vi "StateLED.vi"(0 "Master State":enum16{"Normal", "Climb"}(ring)) -> ()   [LabVIEW 2020]
doc: "This VI manages the apperance of the LEDs. The LED coloration and blink pattern report the robot mode and status. See project documentation for details."
uses:
  drivercommands.vi
  robotoutputs.vi
  driverdata.vi
  refnumbers.vi
  sensordata.vi
  autonomousinfo.vi
  <vilib>/vision/NI_Vision_Development_Module.lvlib
panel:
  in  "Color Sensor Raw Index":i32=44
  in  "Cowl Limit Reverse Index":i32=11
  in  "Turret Limit Forward Index":i32=9
  in  "Turret Limit Reverse Index":i32=8
  in  "Tower Sensor Index":i32=46
  in  "Boolean Sensor Off":u32(colorbox)=16750592
  in  "Boolean Sensor On":u32(colorbox)=6618880
  in  "Indexer Sensor Index":i32=45
  in  "Intaking":u32(colorbox)=16711692
  in  "Firing":u32(colorbox)=61212
  in  "Spinning":u32(colorbox)=16765440
  in  "User Value Choice":u8(slide)=255 step=1 scale=0.0..255.0
  in  "User Saturation Choice":u8(slide)=255 step=1 scale=0.0..255.0
  in  "Pressure Insert":u32(colorbox)=91
  in  "Battery Insert":u32(colorbox)=65282
  in  "Pressure Background":u32(colorbox)=16711680
  in  "Battery Background":u32(colorbox)=16711680
  in  "Pressure LED Length":i32=7
  in  "Battery LED Length":i32=7
  in  "Battery Index":i32
  in  "Pressure Index":i32=49
  in  "Swerve 3 LED Index":i32=27
  in  "Swerve 2 LED Index":i32=28
  in  "Swerve 1 LED Index":i32=29
  in  "Swerve LED Length":i32=1
  in  "Swerve 0 LED Index":i32=26
  in  "Locate LED":bool
  in  "LED Index":i32
  out "User Blue":u8
  out "User Green":u8=255
  out "User Red":u8
  in  "Choose Hue":bool
  in  "User Hue Choice":u8(slide) step=1 scale=0.0..255.0
  in  "Nominal Chase":u32(colorbox)=65280
  in  "Human Player Signal (blink)":u32(colorbox)=65280
  in  "Diverting Power":u32(colorbox)
  in  "Master Caution Chase":u32(colorbox)=16711680
  in  "Autonomous Chase":u32(colorbox)=16727040
  in  "Driving":u32(colorbox)=43263
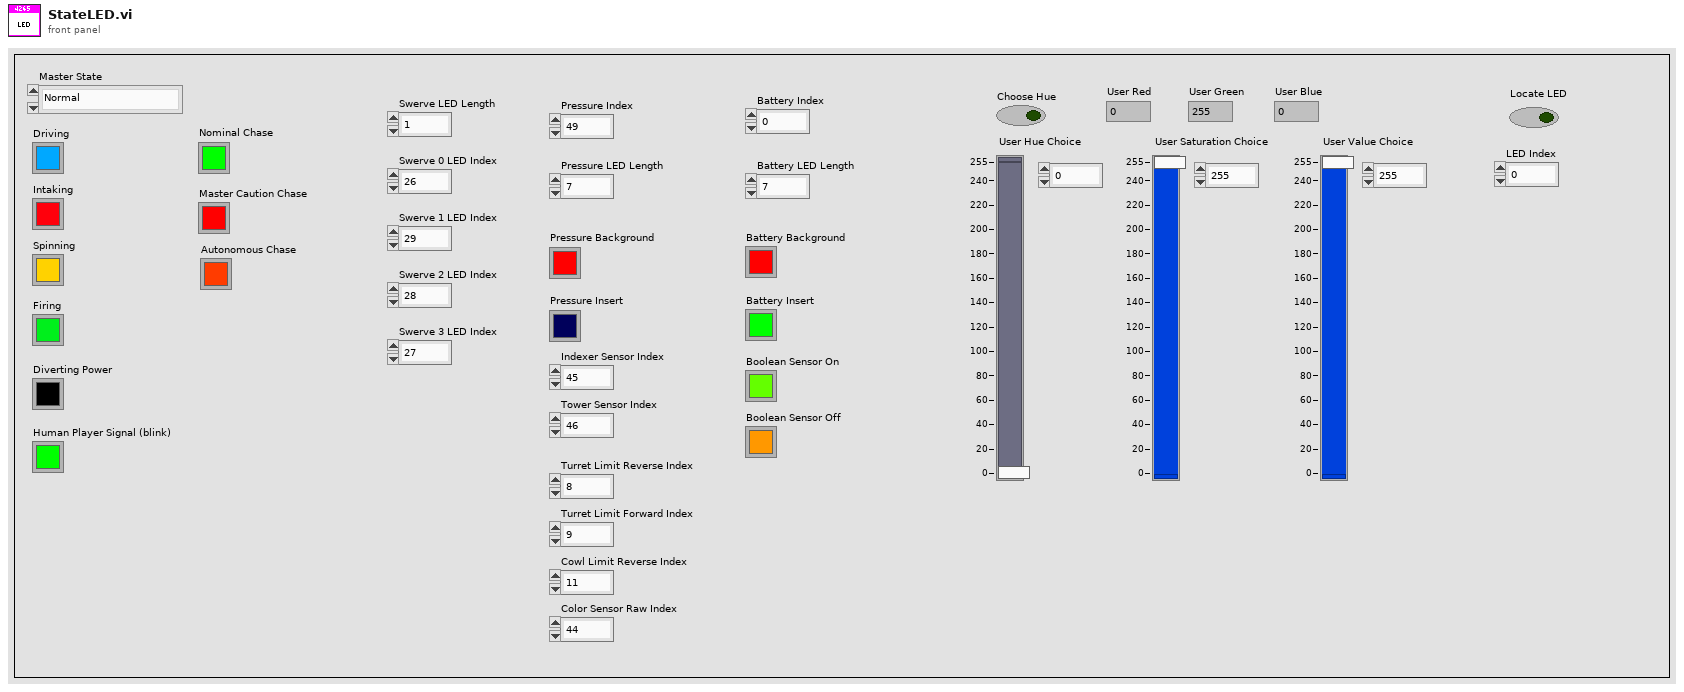
[diagram p1: front panel]
types:
  T1 = enum16{"Normal", "Party Mode", "Choose Hue", "Debug", "Locate LED", "Distance Rainbow"}
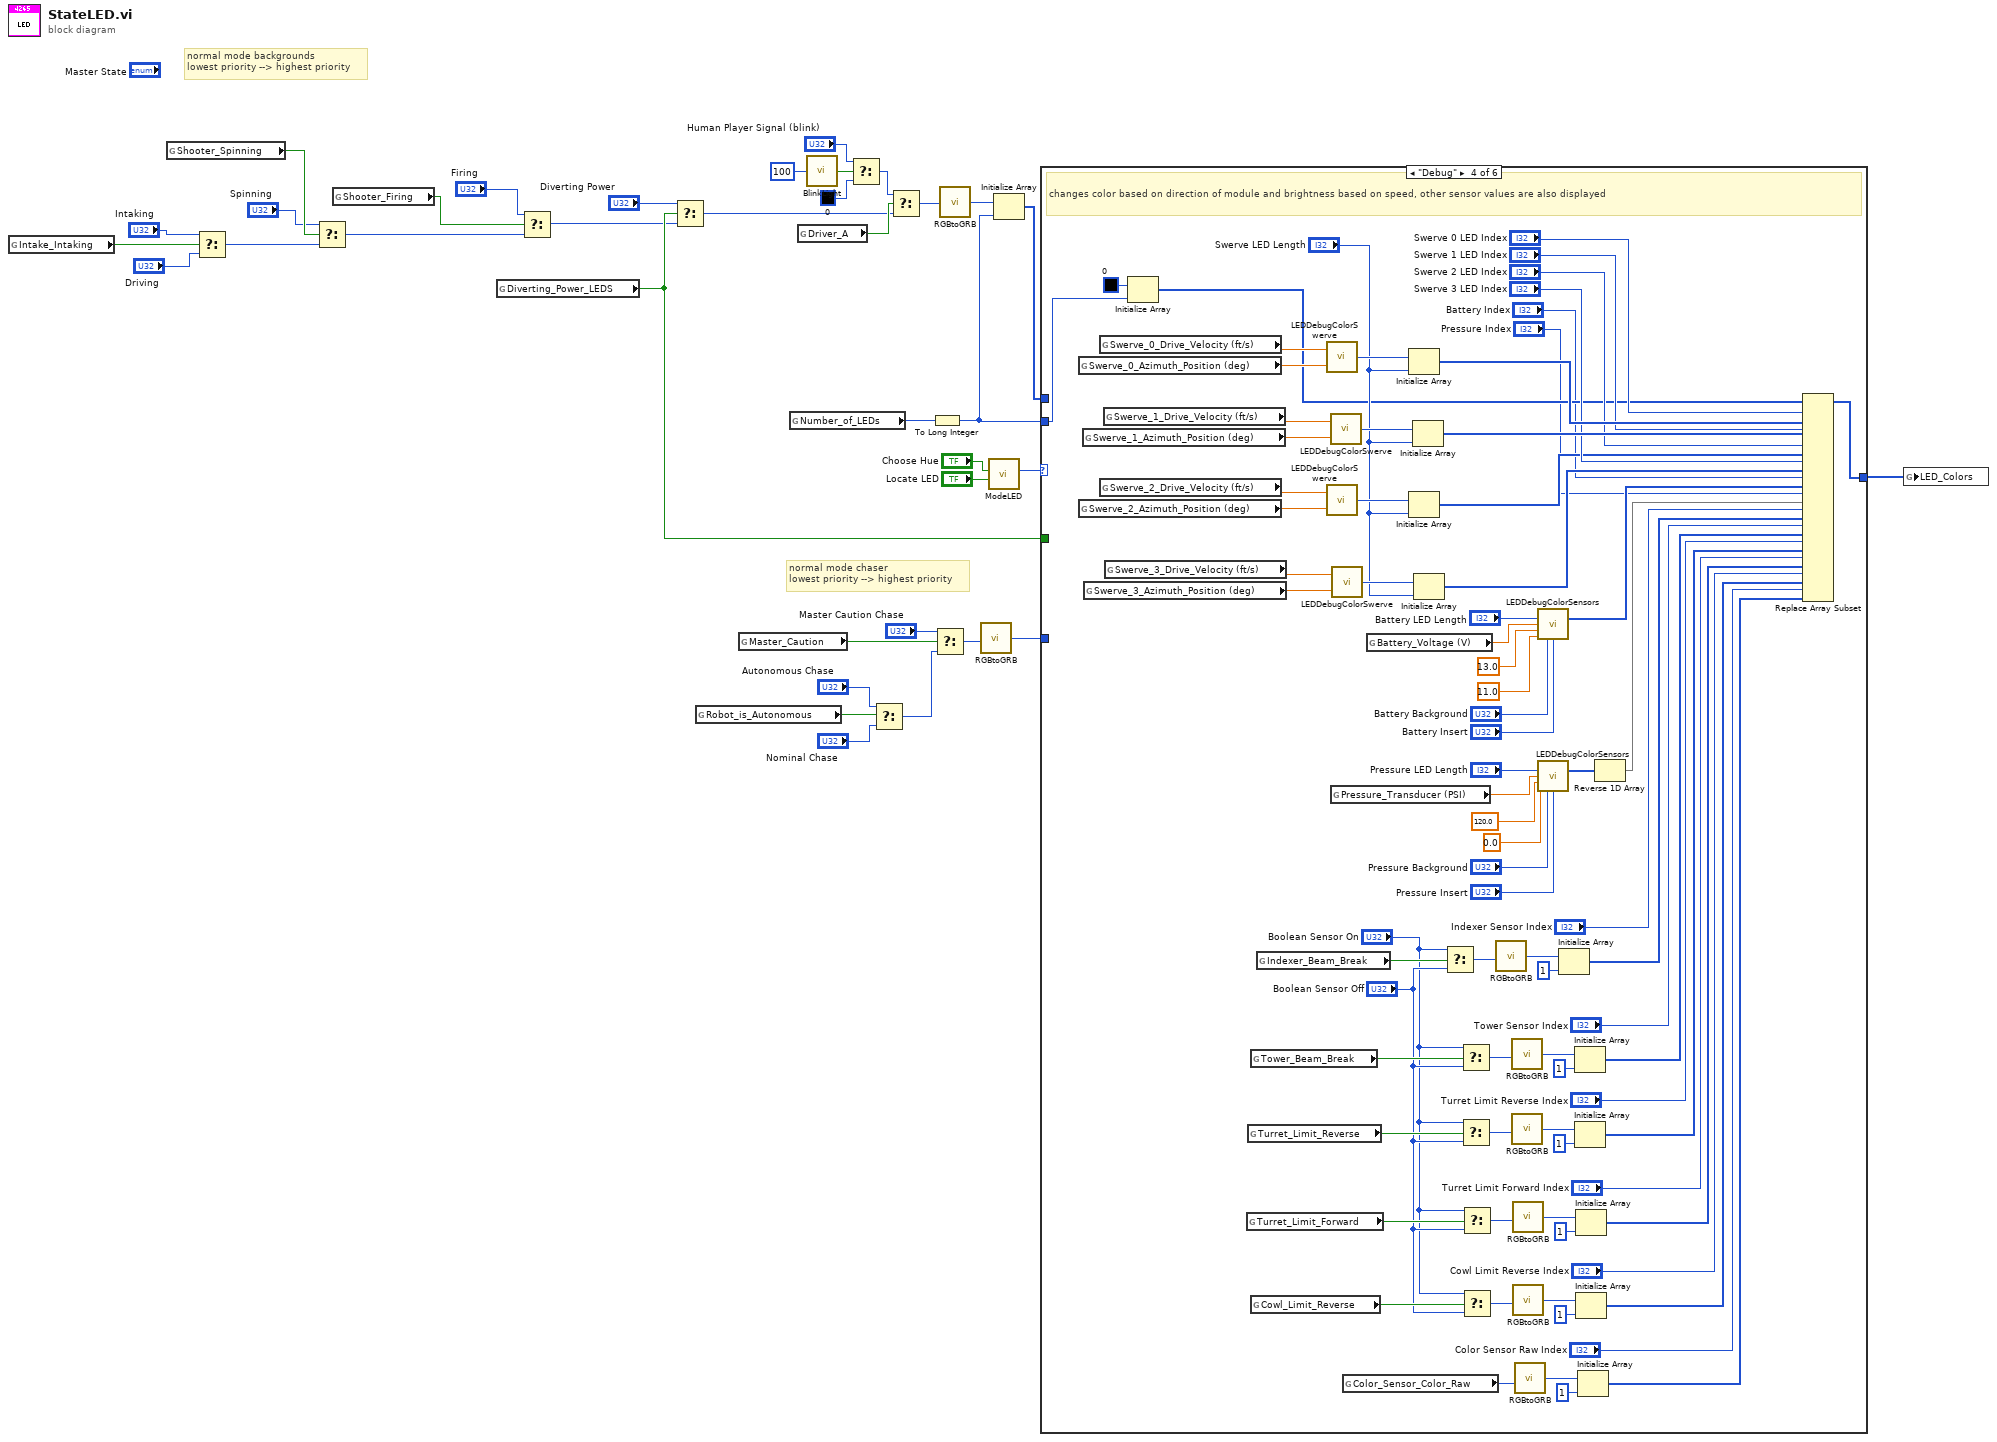
[diagram p0: block diagram]
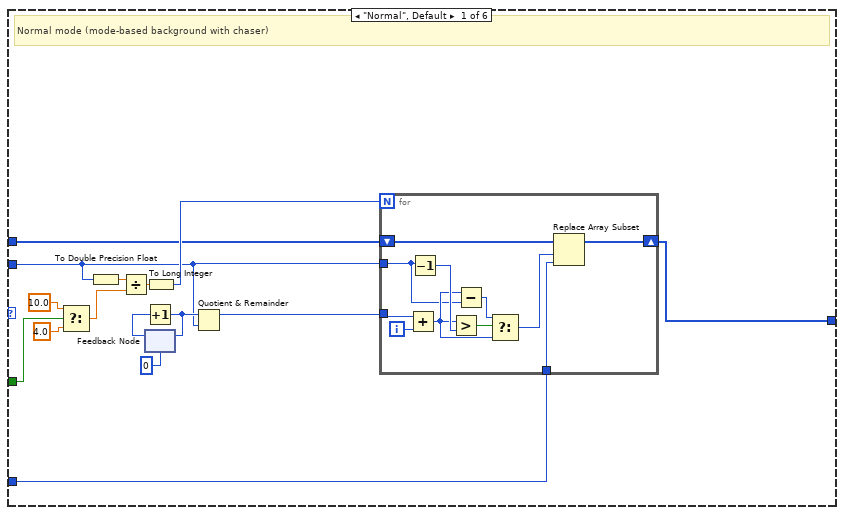
[diagram p2: hidden frame]
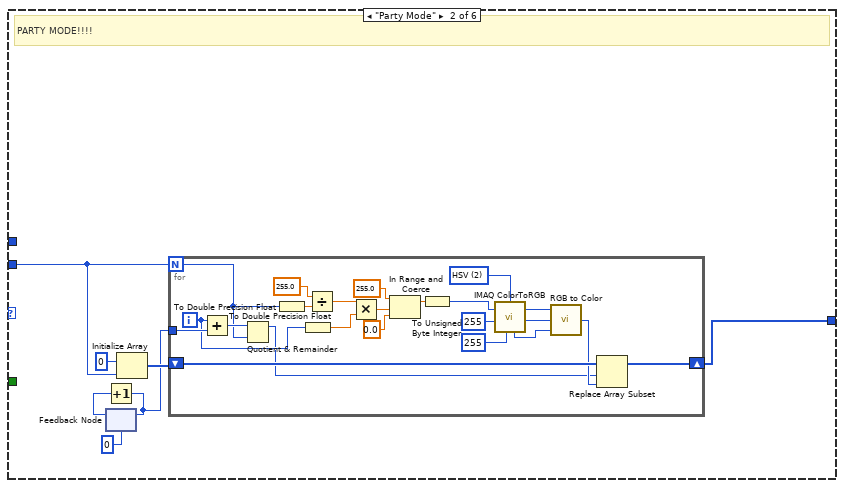
[diagram p3: hidden frame]
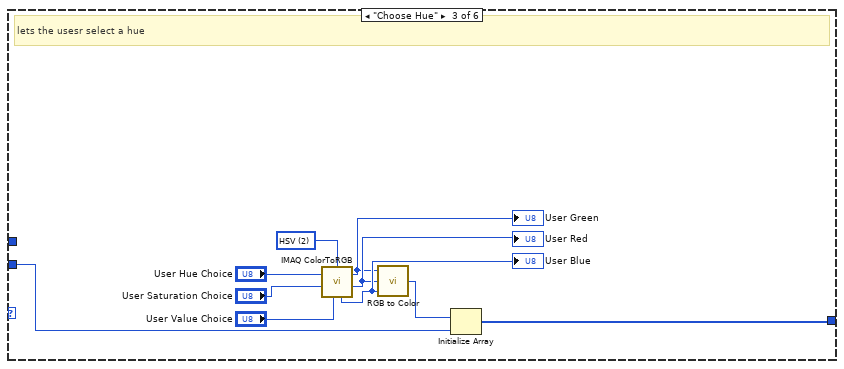
[diagram p4: hidden frame]
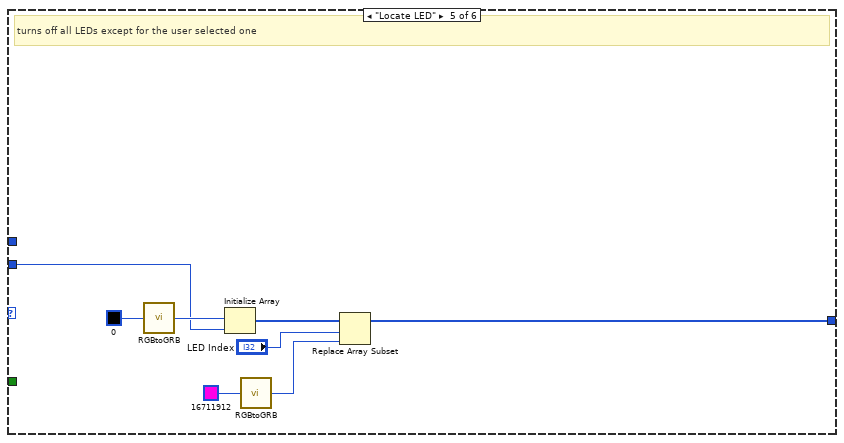
[diagram p5: hidden frame]
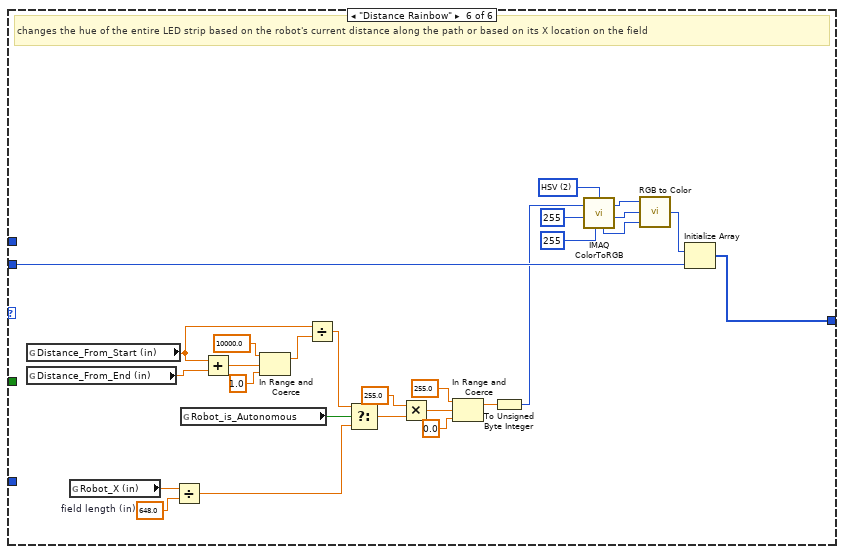
[diagram p6: hidden frame]
diagram:
  # "normal mode chaser\nlowest priority --> highest priority"
  # "normal mode backgrounds\nlowest priority --> highest priority"
  n1 = global read "robotoutputs.vi" "Intake_Intaking"() -> (w4:bool)
  n2 = global read "robotoutputs.vi" "Shooter_Spinning"() -> (w8:bool)
  n3 = Select(t="Intaking", s=w4, f="Driving") -> (s? t:f=w1:u32)
  n4 = Select(t="Spinning", s=w8, f=w1) -> (s? t:f=w6:u32)
  n5 = global read "robotoutputs.vi" "Shooter_Firing"() -> (w3:bool)
  n6 = global read "robotoutputs.vi" "Diverting_Power_LEDS"() -> (w16:bool)
  n7 = Select(t="Firing", s=w3, f=w6) -> (s? t:f=w15:u32)
  n8 = Select(t="Diverting Power", s=w16, f=w15) -> (s? t:f=w30:u32)
  n9 = global read "driverdata.vi" "Robot_is_Autonomous"() -> (w13:bool)
  n10 = global read "driverdata.vi" "Master_Caution"() -> (w25:bool)
  n11 = global read "refnumbers.vi" "Number_of_LEDs"() -> (w9:u16)
  n12 = global read "drivercommands.vi" "Driver_A"() -> (w35:bool)
  n13 = call "BlinkLight.vi"("Blink Interval (ms)"=u32 100) -> ("Blinked Output"=w34:bool)
  n14 = Select(t="Human Player Signal (blink)", s=w34, f=u32 0 ("Color (RGB)")) -> (s? t:f=w31:u32)
  n15 = Select(t="Autonomous Chase", s=w13, f="Nominal Chase") -> (s? t:f=w10:u32)
  n16 = Select(t=w31, s=w35, f=w30) -> (s? t:f=w29:u32)
  n17 = To Long Integer(number=w9) -> (32bit integer=w18:i32)
  n18 = Select(t="Master Caution Chase", s=w25, f=w10) -> (s? t:f=w17:u32)
  n19 = call "RGBtoGRB.vi"("Color (RGB)"=w29) -> ("Color (GRB)"=w28:u32)
  n20 = call "RGBtoGRB.vi"("Color (RGB)"=w17) -> ("Color (GRB)"=w22:u32)
  n21 = call "ModeLED.vi"("Locate LED"="Locate LED", "Choose Hue"="Choose Hue") -> ("LED Mode"=w21:T1)  [unwired: 9 in]
  n22 = Initialize Array(w28, w18) -> (w23:u32[])
  n23 = case shown="\"Debug\"" w21 {
    tunnel: w23 -> [w42 _ _ _ _ _]
    tunnel: [w41 w67 w96 w176 w183 w208] -> w24
    tunnel: w22 -> [w51 _ _ _ _ _]
    tunnel: w18 -> [w43 w64 w95 w159 w182 w209]
    tunnel: w16 -> [w38 _ _ _ _ _]
    frame "Normal", Default {
      # "Normal mode (mode-based background with chaser)"
      n24 = Select(t=10.0, s=w38, f=4.0 ("y")) -> (s? t:f=w39:dbl)
      n25 = To Double Precision Float(number=w43) -> (double precision float=w50:dbl)
      n26 = Divide(x=w50, y=w39) -> (x/y=w49:dbl)
      n27 = feedback #1(0) -> (w47:i32)
      n28 = Increment(x=w47) -> (x+1=w48:i32)
      n29 = feedback-in #1(w48) -> ()
      n30 = To Long Integer(number=w49) -> (32bit integer=w45:i32)
      n31 = Quotient & Remainder(x=w48, y=w43) -> (x-y*floor(x/y)=w44:i32)  [unwired: 1 out]
      n32 = for {
        N: w45 -> [_]
        tunnel: w44 -> [w62]
        tunnel: w43 -> [w53]
        shift-right: [w56] -> w41
        shift-left: w42 -> [w57]
        tunnel: w51 -> [w55]
        i -> [w59]
        n33 = Add(x=w62, y=w59) -> (x+y=w54:i32)
        n34 = Decrement(x=w53) -> (x-1=w61:i32)
        n35 = Greater?(x=w54, y=w61) -> (0:w60:bool)
        n36 = Subtract(x=w54, y=w53) -> (x-y=w52:i32)
        n37 = Select(t=w52, s=w60, f=w54) -> (s? t:f=w58:i32)
        n38 = Replace Array Subset(array=w57, new element=w55, index=w58) -> (w56:u32[])
      }
    }
    frame "Party Mode" {
      # "PARTY MODE!!!!"
      n39 = feedback #2(0) -> (w66:i32)
      n40 = Increment(x=w66) -> (x+1=w63:i32)
      n41 = feedback-in #2(w63) -> ()
      n42 = Initialize Array(u32 0 ("element"), w64) -> (w68:u32[])
      n43 = for {
        N: w64 -> [w72]
        shift-right: [w80] -> w67
        shift-left: w68 -> [w81]
        tunnel: w63 -> [w74]
        i -> [w71]
        w90 = u16 2 items=["RGB", "HSL", "HSV", "HSI"] ("Color Mode")
        n44 = Add(x=w71, y=w74) -> (x+y=w73:i32)
        n45 = Quotient & Remainder(x=w73, y=w72) -> (x-y*floor(x/y)=w70:i32)  [unwired: 1 out]
        n46 = To Double Precision Float(number=w72) -> (double precision float=w89:dbl)
        n47 = To Double Precision Float(number=w71) -> (double precision float=w86:dbl)
        n48 = Divide(x=255.0, y=w89) -> (x/y=w87:dbl)
        n49 = Multiply(x=w87, y=w86) -> (x*y=w85:dbl)
        n50 = In Range and Coerce(upper limit=255.0, x=w85, lower limit=0.0) -> (coerced(x)=w82:dbl)  [unwired: 1 out]
        n51 = To Unsigned Byte Integer(number=w82) -> (unsigned 8bit integer=w75:u8)
        n52 = call "IMAQ ColorToRGB"("Green or Sat value"=u8 255, "Blue or Luma or Val or Inten value"=u8 255, "Red or Hue value"=w75, "Color Mode"=w90) -> ("Blue value"=w76:u8, "Green value"=w77:u8, "Red value"=w78:u8)  [unwired: 1 in, 1 out]
        n53 = call <vilib>:"RGB to Color.vi"("B"=w76, "G"=w77, "R"=w78) -> ("Color"=w79:u32)
        n54 = Replace Array Subset(array=w81, new element=w79, index=w70) -> (w80:u32[])
      }
    }
    frame "Choose Hue" {
      w98 = u16 2 items=["RGB", "HSL", "HSV", "HSI"] ("Color Mode")
      # "lets the usesr select a hue"
      n55 = call "IMAQ ColorToRGB"("Green or Sat value"="User Saturation Choice", "Blue or Luma or Val or Inten value"="User Value Choice", "Red or Hue value"="User Hue Choice", "Color Mode"=w98) -> ("Blue value"=w101:u8, "Green value"=w100:u8, "Red value"=w99:u8)  [unwired: 1 in, 1 out]
      "User Red" <- w100
      "User Green" <- w99
      "User Blue" <- w101
      n56 = call <vilib>:"RGB to Color.vi"("B"=w101, "G"=w100, "R"=w99) -> ("Color"=w97:u32)
      n57 = Initialize Array(w97, w95) -> (w96:u32[])
    }
    frame "Debug" {
      # "changes color based on direction of module and brightness based on speed, other sensor values are also displayed"
      n58 = global read "sensordata.vi" "Swerve_0_Azimuth_Position (deg)"() -> (w180:dbl)
      n59 = global read "sensordata.vi" "Swerve_2_Azimuth_Position (deg)"() -> (w163:dbl)
      n60 = global read "sensordata.vi" "Swerve_1_Azimuth_Position (deg)"() -> (w173:dbl)
      n61 = global read "sensordata.vi" "Swerve_3_Azimuth_Position (deg)"() -> (w166:dbl)
      n62 = global read "sensordata.vi" "Swerve_0_Drive_Velocity (ft/s)"() -> (w181:dbl)
      n63 = global read "sensordata.vi" "Swerve_2_Drive_Velocity (ft/s)"() -> (w165:dbl)
      n64 = global read "sensordata.vi" "Swerve_1_Drive_Velocity (ft/s)"() -> (w175:dbl)
      n65 = global read "sensordata.vi" "Swerve_3_Drive_Velocity (ft/s)"() -> (w168:dbl)
      n66 = Initialize Array(u32 0 ("Color (RGB)"), w159) -> (w157:u32[])
      n67 = global read "sensordata.vi" "Turret_Limit_Forward"() -> (w120:bool)
      n68 = global read "sensordata.vi" "Turret_Limit_Reverse"() -> (w124:bool)
      n69 = global read "sensordata.vi" "Tower_Beam_Break"() -> (w130:bool)
      n70 = global read "sensordata.vi" "Cowl_Limit_Reverse"() -> (w116:bool)
      n71 = global read "sensordata.vi" "Indexer_Beam_Break"() -> (w135:bool)
      n72 = call "LEDDebugColorSwerve.vi"("Azimuth_Angle (deg [-180,180])"=w180, "Drive Velocity (ft/s)"=w181) -> ("Color"=w178:u32)
      n73 = call "LEDDebugColorSwerve.vi"("Azimuth_Angle (deg [-180,180])"=w163, "Drive Velocity (ft/s)"=w165) -> ("Color"=w164:u32)
      n74 = call "LEDDebugColorSwerve.vi"("Azimuth_Angle (deg [-180,180])"=w173, "Drive Velocity (ft/s)"=w175) -> ("Color"=w174:u32)
      n75 = global read "sensordata.vi" "Pressure_Transducer (PSI)"() -> (w144:dbl)
      n76 = call "LEDDebugColorSwerve.vi"("Azimuth_Angle (deg [-180,180])"=w166, "Drive Velocity (ft/s)"=w168) -> ("Color"=w167:u32)
      n77 = global read "sensordata.vi" "Color_Sensor_Color_Raw"() -> (w105:u32)
      n78 = global read "sensordata.vi" "Battery_Voltage (V)"() -> (w156:dbl)
      n79 = Initialize Array(w178, "Swerve LED Length") -> (w177:u32[])
      n80 = Initialize Array(w164, "Swerve LED Length") -> (w161:u32[])
      n81 = Initialize Array(w174, "Swerve LED Length") -> (w172:u32[])
      n82 = Initialize Array(w167, "Swerve LED Length") -> (w160:u32[])
      n83 = Select(t="Boolean Sensor On", s=w135, f="Boolean Sensor Off") -> (s? t:f=w136:u32)
      n84 = Select(t="Boolean Sensor On", s=w130, f="Boolean Sensor Off") -> (s? t:f=w131:u32)
      n85 = Select(t="Boolean Sensor On", s=w124, f="Boolean Sensor Off") -> (s? t:f=w125:u32)
      n86 = Select(t="Boolean Sensor On", s=w120, f="Boolean Sensor Off") -> (s? t:f=w121:u32)
      n87 = Select(t="Boolean Sensor On", s=w116, f="Boolean Sensor Off") -> (s? t:f=w117:u32)
      n88 = call "RGBtoGRB.vi"("Color (RGB)"=w136) -> ("Color (GRB)"=w139:u32)
      n89 = call "RGBtoGRB.vi"("Color (RGB)"=w131) -> ("Color (GRB)"=w133:u32)
      n90 = call "RGBtoGRB.vi"("Color (RGB)"=w125) -> ("Color (GRB)"=w127:u32)
      n91 = call "RGBtoGRB.vi"("Color (RGB)"=w121) -> ("Color (GRB)"=w123:u32)
      n92 = call "RGBtoGRB.vi"("Color (RGB)"=w117) -> ("Color (GRB)"=w119:u32)
      n93 = call "RGBtoGRB.vi"("Color (RGB)"=w105) -> ("Color (GRB)"=w107:u32)
      n94 = call "LEDDebugColorSensors.vi"("LED Length"="Battery LED Length", "Value"=w156, "Max"=13.0, "Min"=11.0, "Background Color"="Battery Background", "Color to Insert"="Battery Insert") -> ("Output Color Array"=w153:u32[])  [unwired: 9 in]
      n95 = call "LEDDebugColorSensors.vi"("LED Length"="Pressure LED Length", "Value"=w144, "Max"=120.0, "Min"=0.0, "Background Color"="Pressure Background", "Color to Insert"="Pressure Insert") -> ("Output Color Array"=w141:u32[])  [unwired: 9 in]
      n96 = Initialize Array(w139, 1 ("dimension size")) -> (w137:u32[])
      n97 = Initialize Array(w133, 1 ("dimension size")) -> (w128:u32[])
      n98 = Initialize Array(w127, 1 ("dimension size")) -> (w112:u32[])
      n99 = Initialize Array(w123, 1 ("dimension size")) -> (w110:u32[])
      n100 = Initialize Array(w119, 1 ("dimension size")) -> (w108:u32[])
      n101 = Initialize Array(w107, 1 ("dimension size")) -> (w103:u32[])
      n102 = Reverse 1D Array(array=w141) -> (reversed array=w140:u32[])
      n103 = Replace Array Subset(array=w157, new element #1=w177, index #1="Swerve 0 LED Index", new element #2=w172, index #2="Swerve 1 LED Index", new element #3=w161, index #3="Swerve 2 LED Index", new element #4=w160, index #4="Swerve 3 LED Index", new element #5=w153, index #5="Battery Index", new element #6=w140, index #6="Pressure Index", new element #7=w137, index #7="Indexer Sensor Index", new element #8=w128, index #8="Tower Sensor Index", new element #9=w112, index #9="Turret Limit Reverse Index", new element #10=w110, index #10="Turret Limit Forward Index", new element #11=w108, index #11="Cowl Limit Reverse Index", new element #12=w103, index #12="Color Sensor Raw Index") -> (w176:u32[])
    }
    frame "Locate LED" {
      # "turns off all LEDs except for the user selected one"
      n104 = call "RGBtoGRB.vi"("Color (RGB)"=u32 0) -> ("Color (GRB)"=w188:u32)
      n105 = Initialize Array(w188, w182) -> (w187:u32[])
      n106 = call "RGBtoGRB.vi"("Color (RGB)"=u32 16711912) -> ("Color (GRB)"=w185:u32)
      n107 = Replace Array Subset(array=w187, new element=w185, index="LED Index") -> (w183:u32[])
    }
    frame "Distance Rainbow" {
      w196 = 648.0  # field length (in)
      w213 = u16 2 items=["RGB", "HSL", "HSV", "HSI"] ("Color Mode")
      # "changes the hue of the entire LED strip based on the robot's current distance along the path or based on its X location on the field"
      n108 = global read "autonomousinfo.vi" "Distance_From_Start (in)"() -> (w202:dbl)
      n109 = global read "autonomousinfo.vi" "Distance_From_End (in)"() -> (w207:dbl)
      n110 = global read "sensordata.vi" "Robot_X (in)"() -> (w197:dbl)
      n111 = Divide(x=w197, y=w196) -> (x/y=w191:dbl)
      n112 = global read "driverdata.vi" "Robot_is_Autonomous"() -> (w190:bool)
      n113 = Add(x=w202, y=w207) -> (x+y=w206:dbl)
      n114 = In Range and Coerce(upper limit=10000.0 ("x"), x=w206, lower limit=1.0) -> (coerced(x)=w203:dbl)  [unwired: 1 out]
      n115 = Divide(x=w202, y=w203) -> (x/y=w201:dbl)
      n116 = Select(t=w201, s=w190, f=w191) -> (s? t:f=w200:dbl)
      n117 = Multiply(x=255.0, y=w200) -> (x*y=w193:dbl)
      n118 = In Range and Coerce(upper limit=255.0 ("x"), x=w193, lower limit=0.0) -> (coerced(x)=w192:dbl)  [unwired: 1 out]
      n119 = To Unsigned Byte Integer(number=w192) -> (unsigned 8bit integer=w198:u8)
      n120 = call "IMAQ ColorToRGB"("Green or Sat value"=u8 255 ("User Saturation Choice 2"), "Blue or Luma or Val or Inten value"=u8 255 ("User Value Choice 2"), "Red or Hue value"=w198, "Color Mode"=w213) -> ("Blue value"=w216:u8, "Green value"=w215:u8, "Red value"=w214:u8)  [unwired: 1 in, 1 out]
      n121 = call <vilib>:"RGB to Color.vi"("B"=w216, "G"=w215, "R"=w214) -> ("Color"=w212:u32)
      n122 = Initialize Array(w212, w209) -> (w208:u32[])
    }
  }
  n123 = global write "robotoutputs.vi" "LED_Colors"(w24) -> ()
